vi "Mosaic_FunctionCall.vi"(6 "Mask":u8[][](array[numeric]), 7 "Current Frame":u8[][](array[numeric]), 8 "error in (no error)":errorcluster, 9 "Running Shift In":dbl[](array[numeric]), 10 "module path":path, 11 "session in":refnum<k35>) -> (0 "error out":errorcluster, 1 "Running Shift Out":dbl[](array[numeric]), 3 "session out":refnum<k35>)   [LabVIEW 2020]
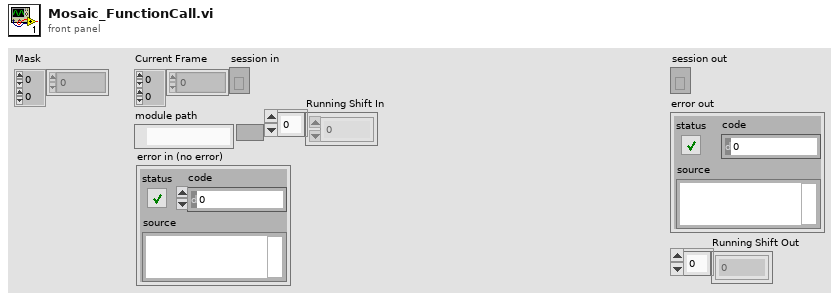
[diagram p1: front panel]
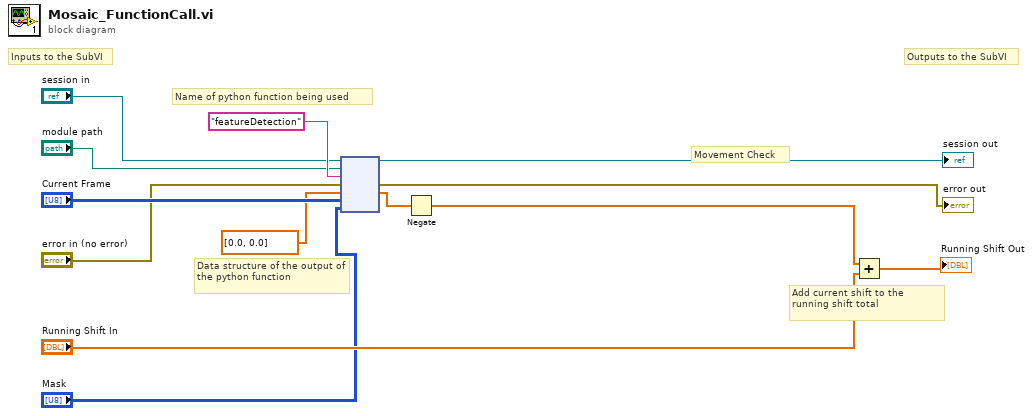
[diagram p0: block diagram]
diagram:
  # "Movement Check"
  # "Outputs to the SubVI"
  # "Add current shift to the running shift total"
  # "Data structure of the output of the python function"
  # "Inputs to the SubVI"
  # "Name of python function being used"
  n1 = node("session in", "module path", "featureDetection" ("function name"), "error in (no error)", dbl[] [0.0, 0.0] ("x"), "Current Frame", "Mask") -> (→"session out":refnum<k35>, →"error out":errorcluster, w3:dbl[])  [unwired: 2 in, 2 out]
  n2 = Negate(x=w3) -> (-x=w2:dbl[])
  n3 = Add(x=w2, y="Running Shift In") -> (x+y=→"Running Shift Out":dbl[])
